vi "Get Current Temp.vi"(8 "error in (no error)":errorcluster, 10 "TempSP":dbl, 11 "Modbus Master in":refnum<class "Modbus Master.lvclass">) -> (0 "error out":errorcluster, 1 "Output (V)":dbl, 2 "Temperature (C)":dbl, 3 "Modbus Master out":refnum<class "Modbus Master.lvclass">)   [LabVIEW 2023, in "PIDModbus.lvlib"]
uses:
  PIDModbus.lvlib
  <vilib>/NI/Modbus Library/API/Master/Modbus Master.lvclass
  Controls/Register Enum.ctl
panel:
  out "Time Elapse":dbl
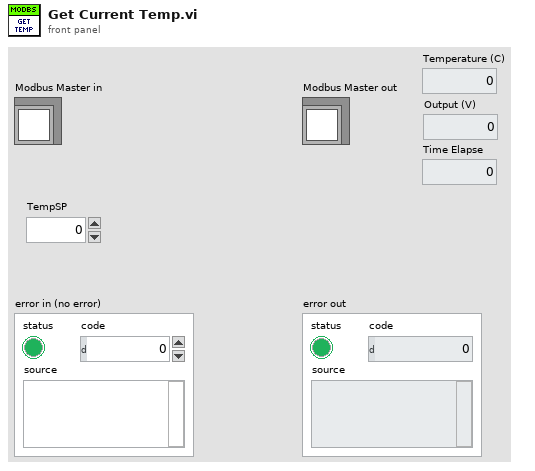
[diagram p1: front panel]
types:
  T1 = typedef "PIDModbus.lvlib/Register Enum.ctl" = u16
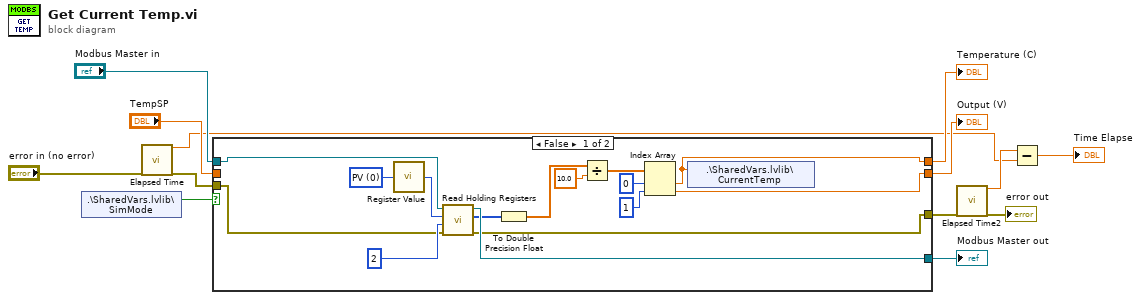
[diagram p0: block diagram]
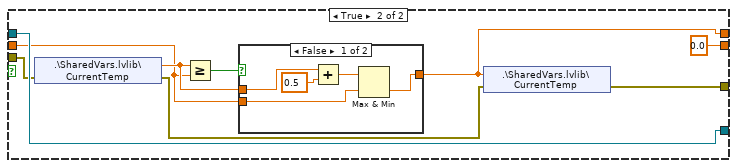
[diagram p2: hidden frame]
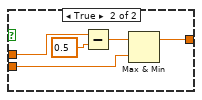
[diagram p3: hidden frame]
diagram:
  n1 = shared-variable ".\\SharedVars.lvlib\\SimMode"() -> (w9:bool)  [unwired: 1 in, 1 out]
  n2 = call "Elapsed Time"("error in (no error)"="error in (no error)") -> ("Present (s)"=w2:dbl, "error out"=w6:errorcluster)  [unwired: 11 in, 6 out]
  n3 = case shown="False" w9 {
    tunnel: [w28 w37] -> w13
    tunnel: w6 -> [w25 w32]
    tunnel: "Modbus Master in" -> [w24 w37]
    tunnel: [w14 w35] -> w11
    tunnel: [w17 0.0] -> w10
    tunnel: [w15 w33] -> w5
    tunnel: "TempSP" -> [_ w29]
    frame False {
      w23 = T1 0 items=["PV"=0, "SV"=5, "P1"=24, "I1"=25, "D1"=26] ("Register")
      n4 = call "Register Value.vi"("Register"=w23) -> ("RegAddr (Hex)"=w22:u16)
      n5 = call-dynamic "Read Holding Registers.vi"("error in"=w25, "number of inputs"=u16 2, "starting address"=w22, "Modbus master in"=w24) -> ("error out"=w15:errorcluster, "register values"=w27:u16[], "Modbus master out"=w28:refnum<class "Modbus Master.lvclass">)  [unwired: 5 in]
      n6 = To Double Precision Float(number=w27) -> (double precision float=w20:dbl[])
      n7 = Divide(x=w20, y=10.0) -> (x/y=w19:dbl[])
      n8 = Index Array(array=w19, index #1=0 ("index"), index #2=1 ("index")) -> (element #1=w14:dbl, element #2=w17:dbl)
      n9 = shared-variable ".\\SharedVars.lvlib\\CurrentTemp"(w14) -> ()  [unwired: 1 in, 1 out]
    }
    frame True {
      n10 = shared-variable ".\\SharedVars.lvlib\\CurrentTemp"(error in=w32) -> (w31:dbl, error out=w34:errorcluster)
      n11 = Greater Or Equal?(x=w31, y=w29) -> (x >= y?=w30:bool)
      n12 = case shown="False" w30 {
        tunnel: [w38 w44] -> w35
        tunnel: w31 -> [w40 w47]
        tunnel: w29 -> [w39 w43]
        frame False {
          n13 = Add(x=w40, y=0.5) -> (x+y=w41:dbl)
          n14 = Max & Min(x=w41, y=w39) -> (min(x,y)=w38:dbl)  [unwired: 1 out]
        }
        frame True {
          n15 = Subtract(x=w47, y=0.5) -> (x-y=w46:dbl)
          n16 = Max & Min(x=w46, y=w43) -> (max(x,y)=w44:dbl)  [unwired: 1 out]
        }
      }
      n17 = shared-variable ".\\SharedVars.lvlib\\CurrentTemp"(w35, error in=w34) -> (error out=w33:errorcluster)
    }
  }
  "Modbus Master out" <- w13
  "Temperature (C)" <- w11
  "Output (V)" <- w10
  n18 = call "Elapsed Time2"("error in (no error)"=w5) -> ("Present (s)"=w3:dbl, "error out"=→"error out":errorcluster)  [unwired: 11 in, 6 out]
  n19 = Subtract(x=w3, y=w2) -> (x-y=→"Time Elapse":dbl)
